vi "DRIVER BINDING UNION MICRO94vi.vi"(4 "Simulazione?":bool) -> ()   [LabVIEW 2019]
doc: "The Basic Serial Read and Write example performs a Serial Port Read, a Serial Port Write, or a combination of these actions. The user selects the actions (read or write) on the front panel. If both are selected, the VI will write the data first, read data, and then close the VISA session that is opened to the port. This VI will wait until the specified number of bytes is received at the port. Only the number of bytes specified will be read.\n\nINSTRUCTIONS:\n1) Select the serial resource and configuration parameters (baud rate, data bits, parity, stop bits, flow control).\n2) Select the operations to be performed. \n3) Connect the serial port to your device. If no device is available, perform a loopback test by doing one of the following. Short pins 2 and 3 on a RS-232 cable or short pin 4 to pin 8 and pin 5 to pin 9 on a RS-485/422 cable. \n4) Run the VI to see the data read. (The \"read string\" will match the \"string to write\" if a loopback test was performed.)\n\nNote: The parameters set for the serial port must match the parameters of the connected instrument or device. In this example, the bytes to read parameter specifies the number of bytes that the serial port reads. If there were more bytes at the port than the number specified in bytes to read, those bytes would not be read. Also, if you specify to read more bytes than the number of bytes actually read, you might receive a timeout error message.\n\nOn the block diagram, the Configure Serial Port VI sets the configuration parameters. The front panel displays the controls used to configure the basic parameters, such as baud rate, data bits, and parity. Constants configure the other parameters the user probably does not need set. After the VISA Configure Serial Port VI opens the VISA session and configures the port, the VI passes the VISA resource name to other VIs that perform operations on that VISA resource. The VISA Write function sends a command to the serial device and the VISA Read function returns data based on the command. The VISA Close function then closes the reference to the serial device. It is important to close the reference; otherwise communication through with that port through protocols other than VISA might not be possible."
uses:
  <vilib>/Utility/file.llb/Read Delimited Spreadsheet (string).vi
  <vilib>/Instr/_visa.llb/VISA Configure Serial Port (Instr).vi
panel:
  out "error in (no error)":errorcluster
  out "error out":errorcluster
  out "String":string
  out "Numeric":i32
  out "Stopped":bool
  out "LOOP TIME (ms)":u32
  out "LETTURA":dbl
  in  "INDIRIZZO":i8
  in  "Ring":u16(ring) items=["RICHIESTA STATO CANALE OPERATIVO", "RICHIESTA PREDISP ALLARME1", "RICHIESTA PREDISP ALLARME2", "RICHIESTA VALORI DI PICCO"]
  in  "delay before read (ms)":u32=500
  in  "flow control":u16(ring) items=["None"=0, "XON/XOFF"=1, "RTS/CTS"=2, "DTR/DSR"=4]
  in  "stop bits":u16(ring)=10 items=["1.0"=10, "1.5"=15, "2.0"=20]
  in  "write":bool=TRUE
  out "string to write":string="*IDN?\r\n"
  in  "read":bool=TRUE
  out "bytes read":u32
  out "read string":string
  in  "parity":u16(ring) items=["None", "Odd", "Even", "Mark", "Space"]
  in  "data bits":u16=8 min=5 max=8 step=1
  in  "baud rate":u32=9600
  in  "VISA resource name":refnum<visa-resource-name>="COM9"
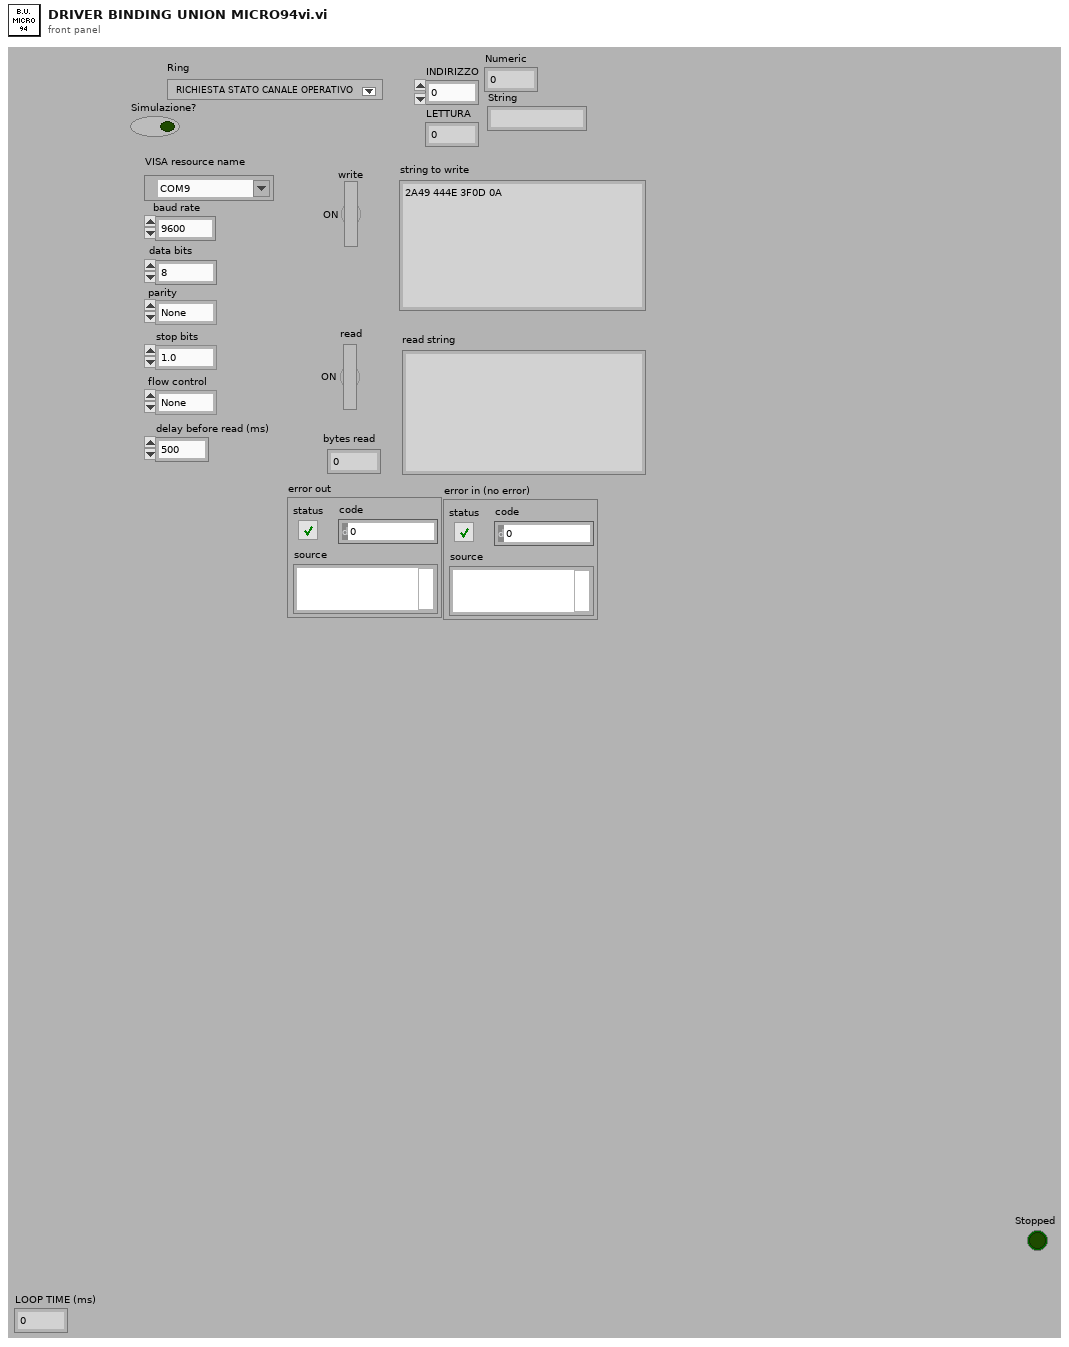
[diagram p1: front panel]
types:
  T1 = cluster{"Array of elements":cluster{"String":string, "variant":variant}[], "Single element":cluster{"String":string, "variant":variant}, "enque at\nopposite end (F)":bool, "no replications (F)":bool}
  T2 = enum16{"ALIGN -CENTER", "ALIGN -TOP LEFT", "ALIGN -AS IS", "ALIGN -CUSTOM"}
  T3 = enum32{"Invalid", "Standard", "Closed", "Hidden", "Minimized", "Maximized"}
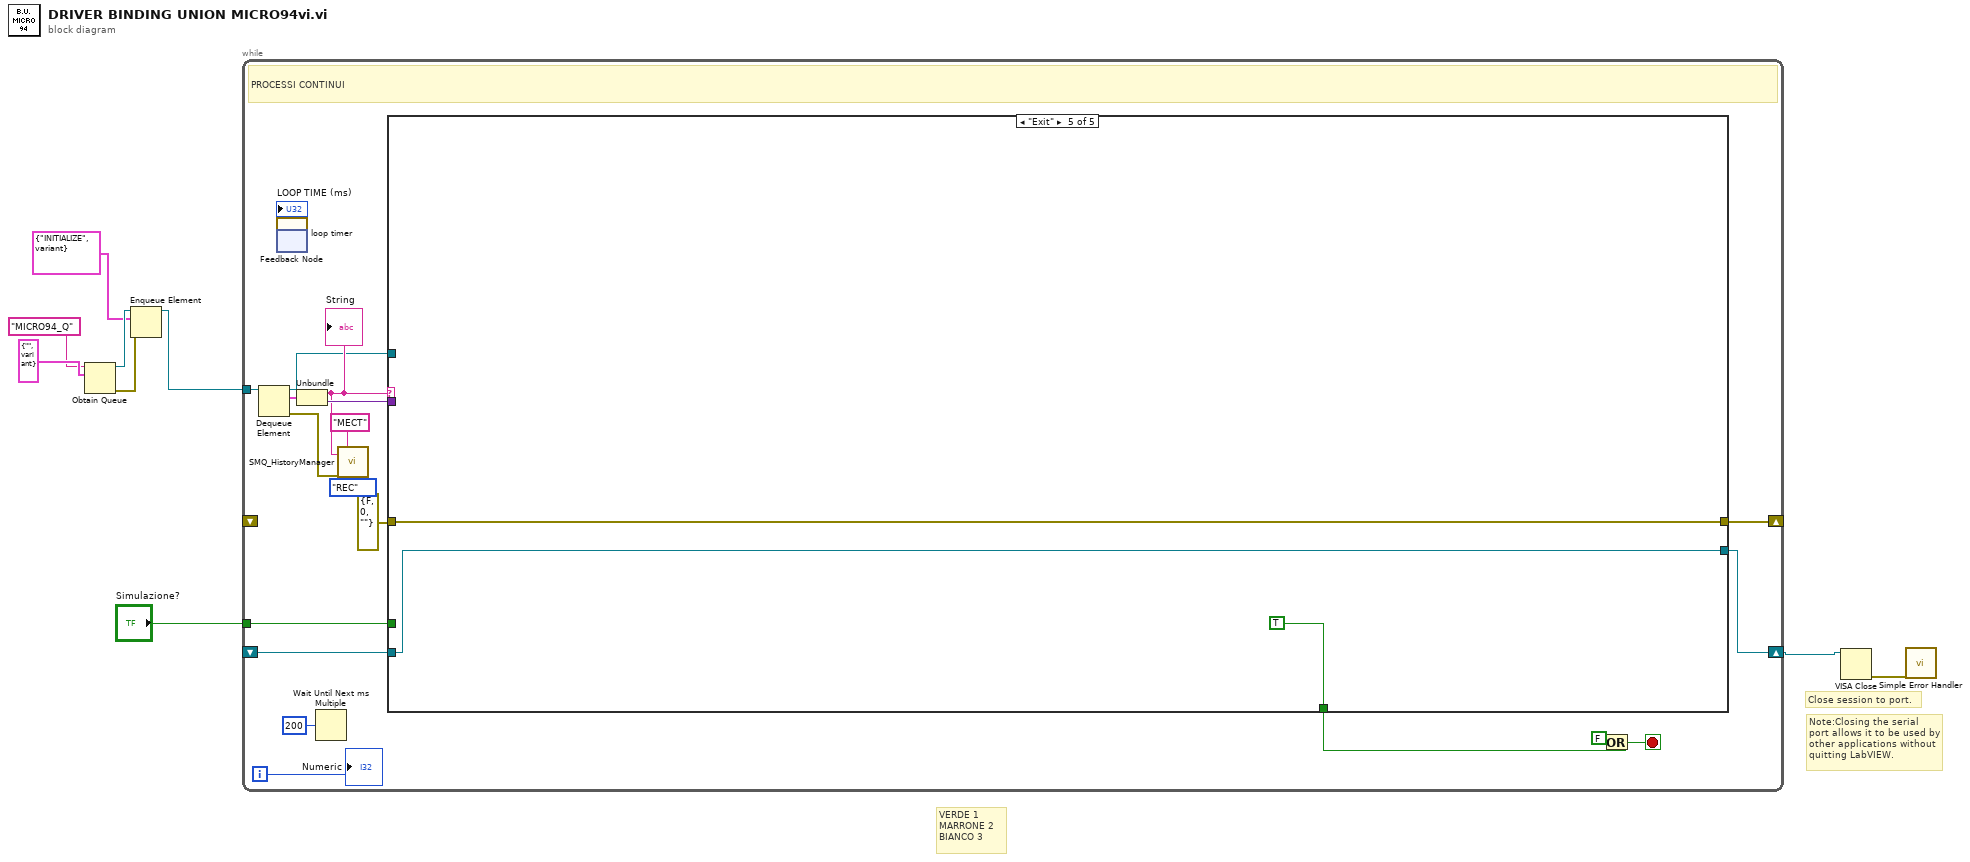
[diagram p0: block diagram]
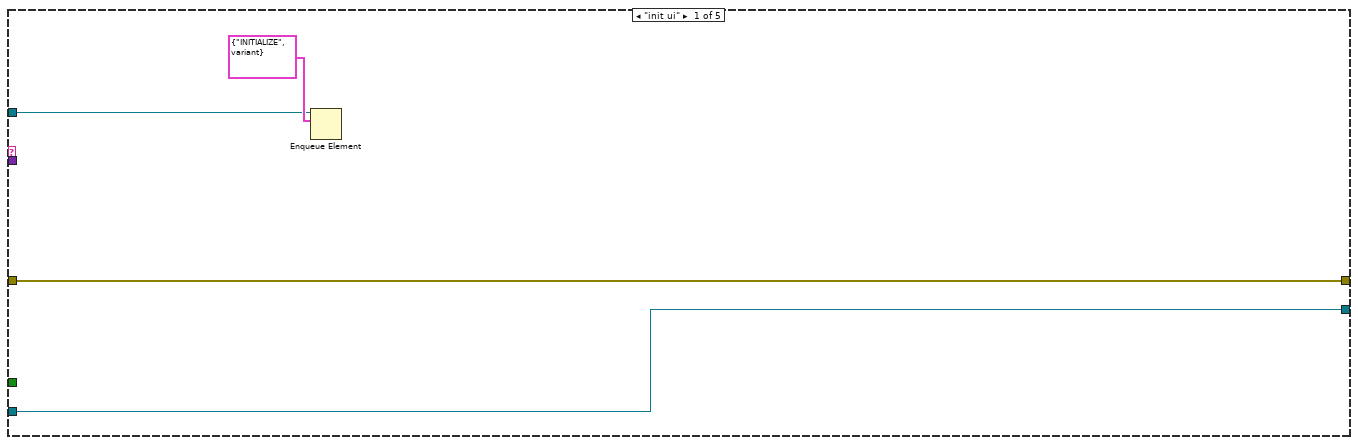
[diagram p2: hidden frame]
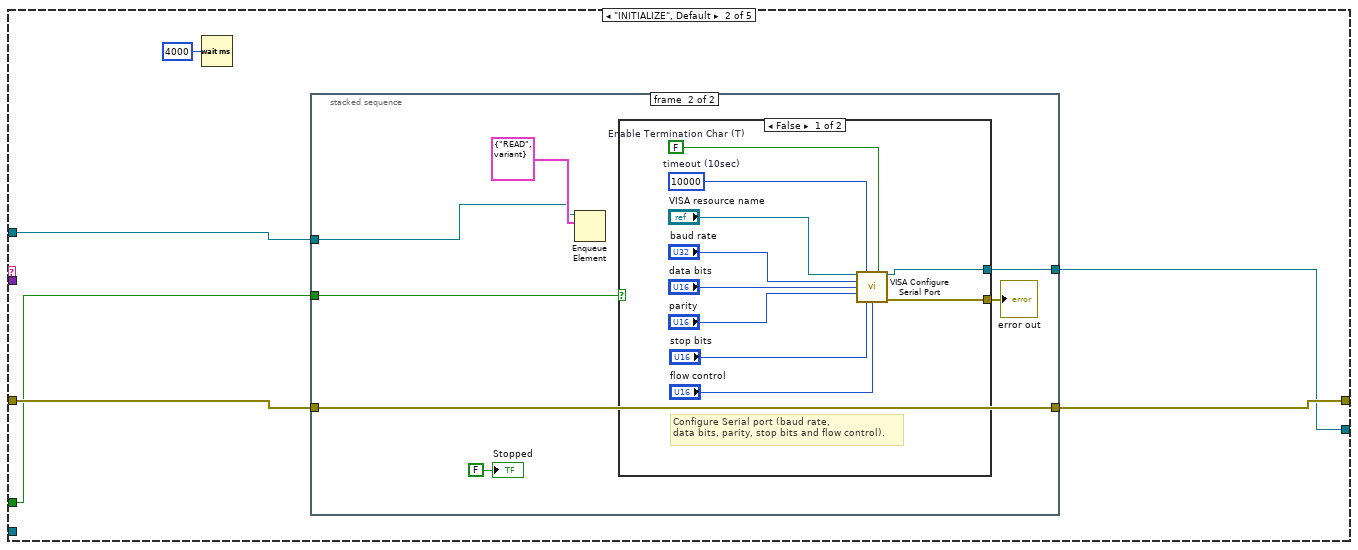
[diagram p3: hidden frame]
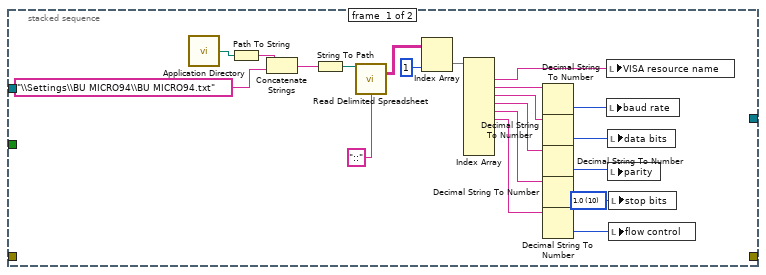
[diagram p4: hidden frame]
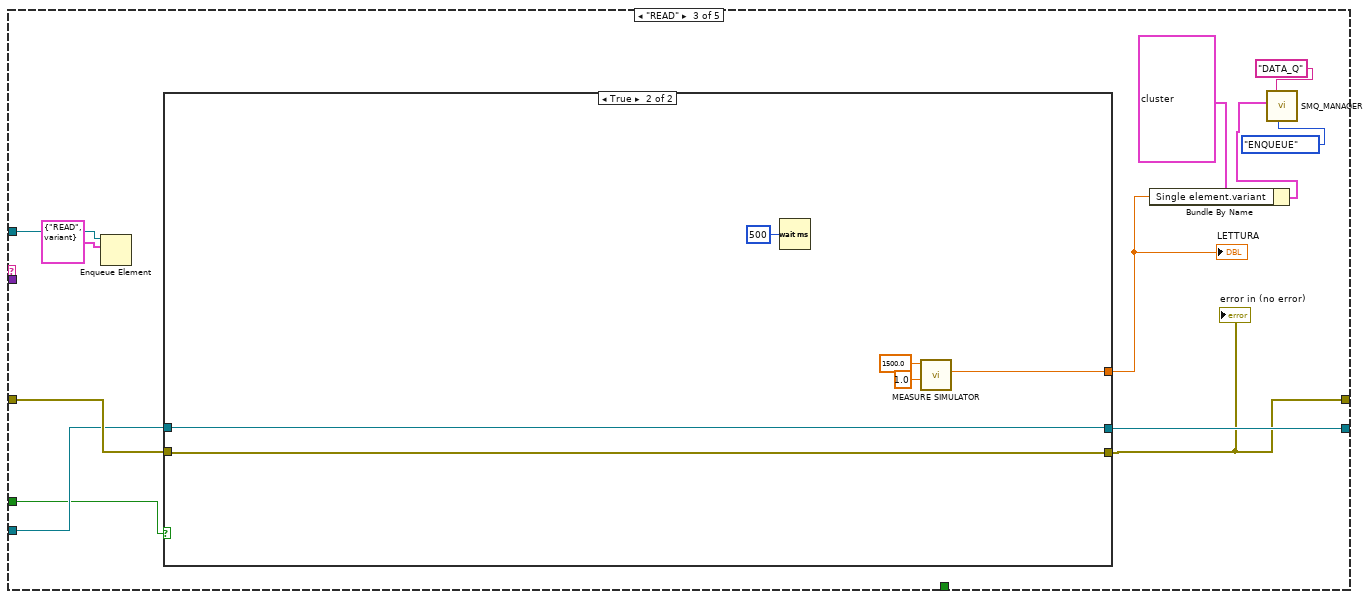
[diagram p6: hidden frame]
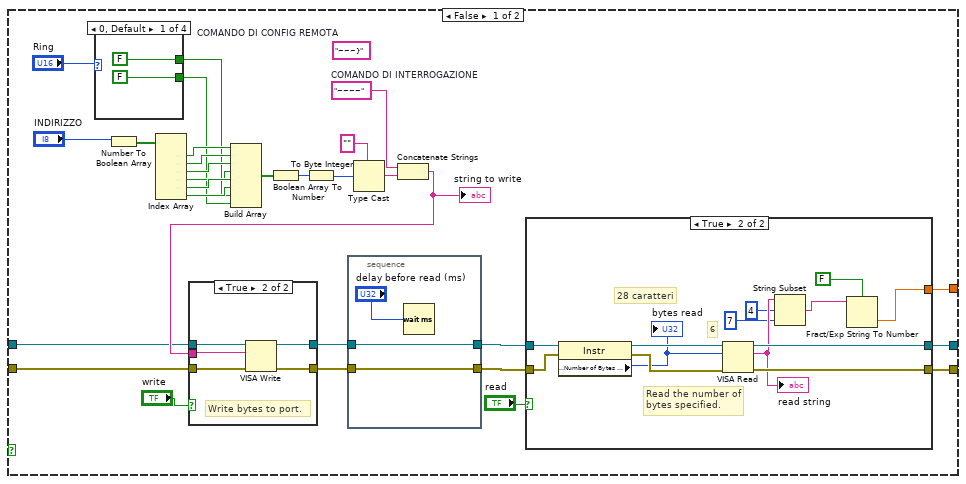
[diagram p7: hidden frame]
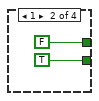
[diagram p8: hidden frame]
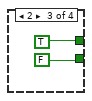
[diagram p9: hidden frame]
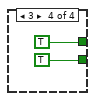
[diagram p10: hidden frame]
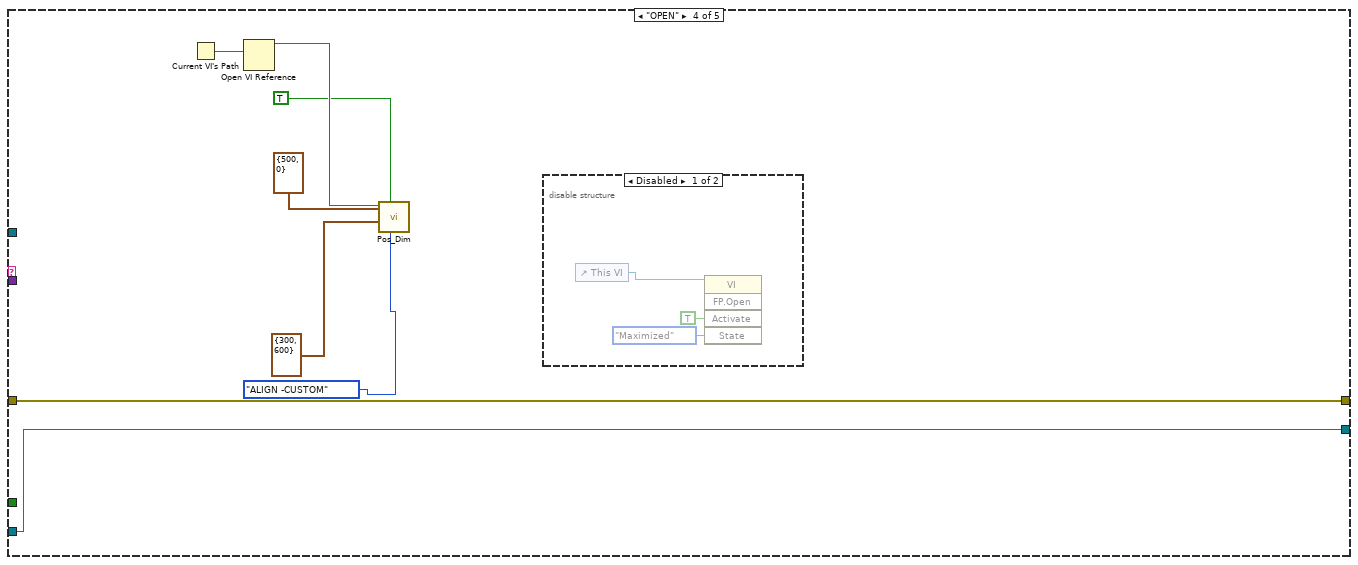
[diagram p13: hidden frame]
diagram:
  # "VERDE 1\nMARRONE 2\nBIANCO 3"
  # "Note:Closing the serial port allows it to be used by other applications without\nquitting LabVIEW."
  # "Close session to port."
  n1 = Obtain Queue(name (unnamed)="MICRO94_Q", element data type=cluster{"String":string, "variant":variant} {"String"="", "variant"=variant} ("element")) -> (queue out=w3:refnum<queue>, error out=w1:errorcluster)  [unwired: 3 in, 1 out]
  n2 = Enqueue Element(queue=w3, element=cluster{"String":string, "variant":variant} {"String"="INITIALIZE", "variant"=variant}, error in (no error)=w1) -> (queue out=w7:refnum<queue>)  [unwired: 1 in, 2 out]
  n3 = while {
    shift-right: [w17] -> _
    shift-left: _ -> [_]
    tunnel: w7 -> [w28]
    shift-right: [w14] -> w8
    shift-left: _ -> [w13]
    tunnel: "Simulazione?" -> [w11]
    i -> [w10]
    stop <- w25 stop-if-true
    # "PROCESSI CONTINUI"
    n4 = Dequeue Element(queue=w28) -> (queue out=w15:refnum<queue>, element=w27:cluster{"String":string, "variant":variant}, error out=w22:errorcluster)  [unwired: 2 in, 1 out]
    n5 = feedback #1() -> (w19:u32)  [unwired: 1 in]
    n6 = call <userlib>:"loop timer.vi"("millisecond timer IN"=w19) -> ("millisecond timer OUT"=w20:u32, "LOOP TIME (ms)"=→"LOOP TIME (ms)":u32)  [unwired: 9 in]
    n7 = feedback-in #1(w20) -> ()
    n8 = Unbundle(w27) -> ("String"=w23:string, "variant"=w26:variant)
    "String" <- w23
    n9 = Wait Until Next ms Multiple(millisecond multiple=u32 200) -> ()  [unwired: 1 out]
    n10 = call <userlib>:"SMQ_HistoryManager.vi"("Caller VI"="MECT", "State"=w23, "error in (no error)"=w22, "Function"=enum16{"INITIALIZE", "REC", "STOP"}."REC") -> ()  [unwired: 14 in, 2 out]
    n11 = case shown="\"Exit\"" w23 {
      tunnel: [_ _ _ _ TRUE] -> w29
      tunnel: errorcluster {"status"=FALSE, "code"=0, "source"=""} ("error in (no error)") -> [w34 w40 w87 w166 w171]
      tunnel: [w34 w39 w83 w166 w171] -> w17
      tunnel: w26 -> [_ _ _ _ _]
      tunnel: w15 -> [w32 w38 w88 _ _]
      tunnel: [w31 w37 w85 w165 w170] -> w14
      tunnel: w13 -> [w31 _ w86 w165 w170]
      tunnel: w11 -> [_ w36 w84 _ _]
      frame "init ui" {
        n12 = Enqueue Element(queue=w32, element=cluster{"String":string, "variant":variant} {"String"="INITIALIZE", "variant"=variant}) -> ()  [unwired: 2 in, 3 out]
      }
      frame "INITIALIZE", Default {
        n13 = Wait (ms)(milliseconds to wait=u32 4000) -> ()  [unwired: 1 out]
        n14 = stacked-sequence {
          tunnel: w40 -> [_ w66]
          tunnel: [_ w66] -> w39
          tunnel: w38 -> [_ w64]
          tunnel: [_ w63] -> w37
          tunnel: w36 -> [_ w62]
          frame #0 {
            w60 = u16 10 items=["1.0"=10, "1.5"=15, "2.0"=20] ("stop bits")
            n15 = call <vilib>:"Application Directory.vi"() -> ("Application Directory"=w42:path)
            n16 = Path To String(path=w42) -> (string=w43:string)
            n17 = Concatenate Strings(w43, "\\Settings\\BU MICRO94\\BU MICRO94.txt" ("string")) -> (w45:string)
            n18 = String To Path(string=w45) -> (path=w46:path)
            n19 = call-poly <vilib>:"Read Delimited Spreadsheet.vi"("file path (dialog if empty)"=w46, "delimiter (\\t)"="::" ("delimiter (\\t)")) -> ("all rows"=w47:string[][])  [unwired: 8 in, 5 out]
            n20 = Index Array(array=w47, index (col)=1 ("disabled index (col)")) -> (element=w49:string[])  [unwired: 1 in]
            n21 = Index Array(array=w49) -> (element #1=w50:string, element #2=w51:string, element #3=w53:string, element #4=w55:string, element #5=w56:string, element #6=w58:string)  [unwired: 10 in, 4 out]
            n22 = Decimal String To Number(string=w51) -> (number=w52:i32)  [unwired: 2 in, 1 out]
            n23 = Decimal String To Number(string=w53) -> (number=w54:i32)  [unwired: 2 in, 1 out]
            n24 = Decimal String To Number(string=w55) -> (number=w57:i32)  [unwired: 2 in, 1 out]
            n25 = Decimal String To Number(string=w56) -> ()  [unwired: 2 in, 2 out]
            n26 = Decimal String To Number(string=w58) -> (number=w59:i32)  [unwired: 2 in, 1 out]
            n27 = local write "VISA resource name"(w50) -> ()
            n28 = local write "baud rate"(w52) -> ()
            n29 = local write "data bits"(w54) -> ()
            n30 = local write "parity"(w57) -> ()
            n31 = local write "stop bits"(w60) -> ()
            n32 = local write "flow control"(w59) -> ()
          }
          frame #1 {
            n33 = Enqueue Element(queue=w64, element=cluster{"String":string, "variant":variant} {"String"="READ", "variant"=variant}) -> ()  [unwired: 2 in, 3 out]
            n34 = case shown="False" w62 {
              tunnel: [w69 _] -> w63
              tunnel: [w68 _] -> w61
              frame False {
                w74 = FALSE  # Enable Termination Char (T)
                w73 = u32 10000  # timeout (10sec)
                # "Configure Serial port (baud rate,\ndata bits, parity, stop bits and flow control)."
                n35 = call-poly "VISA Configure Serial Port"("VISA resource name"="VISA resource name", "timeout (10sec)"=w73, "Enable Termination\nChar (T)"=w74, "baud rate (9600)"="baud rate", "data bits (8)"="data bits", "parity (0:none)"="parity", "stop bits (10: 1 bit)"="stop bits", "flow control (0:none)"="flow control") -> ("VISA resource name out"=w69:refnum<visa-resource-name>, "error out"=w68:errorcluster)  [unwired: 1 in, 5 out]
              }
              frame True {
              }
            }
            "error out" <- w61
            "Stopped" <- FALSE ("Stop")
          }
        }
      }
      frame "READ" {
        n36 = Enqueue Element(queue=w88, element=cluster{"String":string, "variant":variant} {"String"="READ", "variant"=variant}) -> ()  [unwired: 2 in, 3 out]
        n37 = case shown="True" w84 {
          tunnel: [w118 w158] -> w79
          tunnel: w87 -> [w93 w154]
          tunnel: w86 -> [w92 w155]
          tunnel: [w91 w155] -> w85
          tunnel: [w90 w154] -> w83
          frame False {
            (unwired) "~~~}"  # COMANDO DI CONFIG REMOTA
            w109 = "~~~~"  # COMANDO DI INTERROGAZIONE
            n38 = case shown="0, Default" "Ring" {
              tunnel: [FALSE ("element") FALSE ("element") TRUE ("element") TRUE ("element")] -> w103
              tunnel: [FALSE ("element") TRUE ("element") FALSE ("element") TRUE ("element")] -> w104
              frame 0, Default {
              }
              frame 1 {
              }
              frame 2 {
              }
              frame 3 {
              }
            }
            n39 = Number To Boolean Array(number="INDIRIZZO") -> (Boolean array=w101:bool[])
            n40 = Index Array(array=w101) -> (element #1=w111:bool, element #2=w112:bool, element #3=w113:bool, element #4=w114:bool, element #5=w115:bool, element #6=w116:bool)  [unwired: 6 in]
            n41 = Build Array(w111, w112, w113, w114, w115, w116, w103, w104) -> (w117:bool[])
            n42 = Boolean Array To Number(Boolean array=w117) -> (number=w105:u32)
            n43 = To Byte Integer(number=w105) -> (8bit integer=w106:i8)
            n44 = Type Cast(type="", x=w106) -> (*(type *) &x=w108:string)
            n45 = Concatenate Strings(w109, w108) -> (w110:string)
            "string to write" <- w110
            n46 = case shown="True" "write" {
              tunnel: [w131 w136] -> w96
              tunnel: w92 -> [w130 w135]
              tunnel: w93 -> [w131 w134]
              tunnel: [w130 w133] -> w98
              tunnel: w110 -> [_ w132]
              frame False {
              }
              frame True {
                # "Write bytes to port."
                n47 = VISA Write(VISA resource name=w135, write buffer=w132, error in (no error)=w134) -> (VISA resource name out=w133:refnum<visa-resource-name>, error out=w136:errorcluster)  [unwired: 1 out]
              }
            }
            n48 = stacked-sequence {
              tunnel: w96 -> [w129]
              tunnel: [w129] -> w97
              tunnel: w98 -> [w128]
              tunnel: [w128] -> w99
              frame #0 {
                n49 = Wait (ms)(milliseconds to wait="delay before read (ms)") -> ()  [unwired: 1 out]
              }
            }
            n50 = case shown="True" "read" {
              tunnel: w97 -> [w138 w148]
              tunnel: [w138 w152] -> w90
              tunnel: [w139 w151] -> w91
              tunnel: w99 -> [w139 w150]
              tunnel: [nan w140] -> w118
              frame False {
              }
              frame True {
                # "28 caratteri"
                # "6"
                # "Read the number of bytes specified."
                n51 = property class="Instr"(reference=w150, error in=w148) -> (reference out=w149:refnum<visa-resource-name>, error out=w147:errorcluster, "Serial Settings:Number of Bytes at Serial Port"=w146:u32)
                "bytes read" <- w146
                n52 = VISA Read(VISA resource name=w149, byte count=w146, error in (no error)=w147) -> (VISA resource name out=w151:refnum<visa-resource-name>, read buffer=w145:string, error out=w152:errorcluster)  [unwired: 1 out]
                "read string" <- w145
                n53 = String Subset(string=w145, offset (0)=4, length (rest)=7 ("length (rest)")) -> (substring=w142:string)
                n54 = Fract/Exp String To Number(use system decimal point (T)=FALSE, string=w142) -> (number=w140:dbl)  [unwired: 3 out]
              }
            }
          }
          frame True {
            n55 = Wait (ms)(milliseconds to wait=u32 500) -> ()  [unwired: 1 out]
            n56 = call <userlib>:"MEASURE SIMULATOR.vi"("precision %"=1.0, "amplitude"=1500.0) -> ("value"=w158:dbl)  [unwired: 9 in]
          }
        }
        "LETTURA" <- w79
        "error in (no error)" <- w83
        n57 = Bundle By Name(cluster=T1 {"Array of elements"=[], "Single element"={"String"="READ RPM", "variant"=variant}, "enque at\nopposite end (F)"=FALSE, "no replications (F)"=FALSE} ("Enqueue cluster"), "Single element.variant"=w79) -> (w78:T1)
        n58 = call <userlib>:"SMQ_MANAGER.vi"("Function"=enum16{"INITIALIZE", "ENQUEUE", "STOP ALL"}."ENQUEUE", "Queue name"="DATA_Q", "Enqueue cluster"=w78) -> ()  [unwired: 8 in, 1 out]
      }
      frame "OPEN" {
        n59 = Current VI's Path() -> (path=w163:path)
        n60 = Open VI Reference(vi path=w163) -> (vi reference=w164:refnum<vi>)  [unwired: 1 in, 5 out]
        n61 = call "Pos_Dim.vi"("Mode"=T2."ALIGN -CUSTOM", "Open FP"=TRUE, "Size"=cluster{"right":i16, "bottom":i16} {"right"=300, "bottom"=600}, "Poistion"=cluster{"left":i16, "top":i16} {"left"=500, "top"=0}, "VIRefNum  IN"=w164) -> ()  [unwired: 2 in, 5 out]
        n62 = disable-structure shown="Disabled" {
          frame Disabled {
            n63 = control-ref of="This VI"() -> (w167:refnum<vi>)
            n64 = invoke class="VI" method="FP.Open"(reference=w167, "Activate"=TRUE ("Activate?"), "State"=T3."Maximized") -> ()  [unwired: 2 in, 5 out]
          }
          frame Enabled {
          }
        }
      }
      frame "Exit" {
      }
    }
    n65 = Or(x=FALSE, y=w29) -> (x .or. y?=w25:bool)
    "Numeric" <- w10
  }
  n66 = VISA Close(VISA resource name=w8) -> (error out=w9:errorcluster)  [unwired: 1 in]
  n67 = call <vilib>:"Simple Error Handler.vi"("error in (no error)"=w9) -> ()  [unwired: 1 in, 8 out]
